vi "Mouse Down QUEUE.vi"(6 "timeout in ms (-1)":i32, 7 "Operation":T1, 8 "error in":errorcluster, 11 "Ref In":refnum<vi>) -> (0 "error out":errorcluster, 3 "Ref Out":refnum<vi>)   [LabVIEW 2012]
uses:
  Controls/Ref Memory Operations.ctl
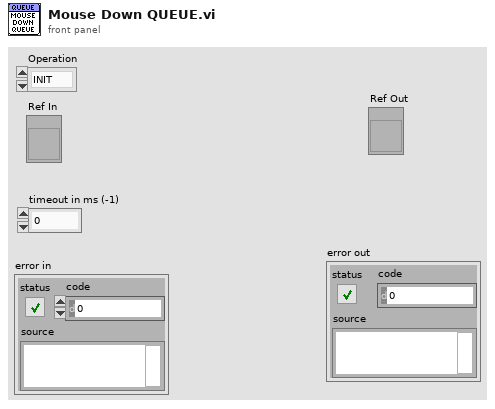
[diagram p1: front panel]
types:
  T1 = typedef "Ref Memory Operations.ctl" = enum16{"INIT", "WRITE", "READ"}
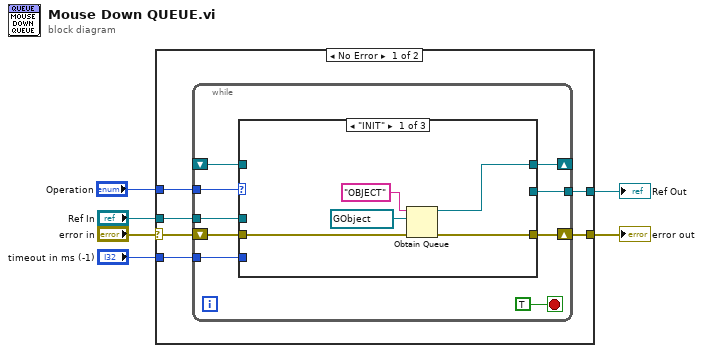
[diagram p0: block diagram]
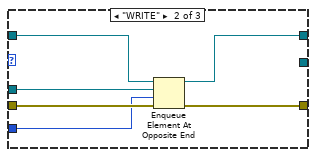
[diagram p2: hidden frame]
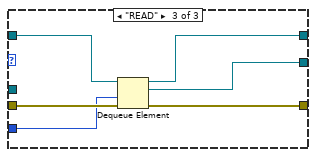
[diagram p3: hidden frame]
diagram:
  n1 = case shown="No Error" "error in" {
    selector: "error in" -> [w9 w39]
    tunnel: "Operation" -> [w12 _]
    tunnel: "Ref In" -> [w11 _]
    tunnel: [w10 w39] -> w4
    tunnel: [w8 _] -> w2
    tunnel: "timeout in ms (-1)" -> [w7 _]
    frame No Error {
      n2 = while {
        tunnel: w12 -> [w20]
        tunnel: w11 -> [w19]
        shift-right: [w18] -> _
        shift-left: _ -> [w17]
        shift-right: [w16] -> w10
        shift-left: w9 -> [w15]
        tunnel: [w14] -> w8
        tunnel: w7 -> [w13]
        stop <- TRUE stop-if-true
        n3 = case shown="\"INIT\"" w20 {
          tunnel: w19 -> [_ w32 _]
          tunnel: [w25 w31 w37] -> w18
          tunnel: w17 -> [_ w30 w38]
          tunnel: [w23 w29 w35] -> w16
          tunnel: w15 -> [w24 w28 w36]
          tunnel: [_ _ w34] -> w14
          tunnel: w13 -> [_ w27 w33]
          frame "INIT" {
            n4 = Obtain Queue(name (unnamed)="OBJECT", element data type=refnum<vi> refnum ("element"), error in (no error)=w24) -> (queue out=w25:refnum<queue>, error out=w23:errorcluster)  [unwired: 2 in, 1 out]
          }
          frame "WRITE" {
            n5 = Enqueue Element At Opposite End(queue=w30, element=w32, timeout in ms (-1)=w27, error in (no error)=w28) -> (queue out=w31:refnum<queue>, error out=w29:errorcluster)  [unwired: 1 out]
          }
          frame "READ" {
            n6 = Dequeue Element(queue=w38, timeout in ms (-1)=w33, error in (no error)=w36) -> (queue out=w37:refnum<queue>, element=w34:refnum<vi>, error out=w35:errorcluster)  [unwired: 1 out]
          }
        }
      }
    }
    frame Error {
    }
  }
  "error out" <- w4
  "Ref Out" <- w2
